vi "SaveTemplatePathToINI.vi"(11 "Template":refnum<class "MetaDataObj.lvclass">) -> ()   [LabVIEW 2016, in "NI_NPW_Project Copying.lvlib"]
uses:
  <resource>/dialog/NewProjectWizard/Project Copying/NI_NPW_Project Copying.lvlib
  <resource>/dialog/NewProjectWizard/MetaDataObj/MetaDataObj.lvclass
  <vilib>/Utility/error.llb/whitespace.ctl
  <resource>/dialog/NewProjectWizard/MetaDataObj/Accessors/Read LocationPath.vi
  <resource>/dialog/NewProjectWizard/MetaDataObj/Accessors/Read Title.vi
  <resource>/dialog/lvconfig.llb/LV Config Read Numeric (I32).vi
panel:
  in  "NewProj.maxNum":string="NewProj.maxNum"
  in  "TemplateTitlesKey":string="NewProj.RecentTitles"
  in  "maxNum Default":i32=10
  in  "TemplatePathsKey":string="NewProj.RecentLocationPaths"
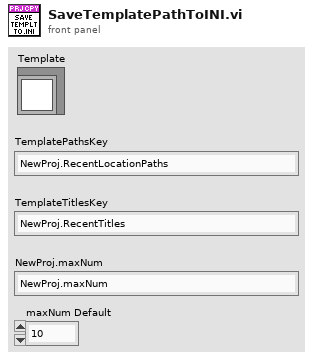
[diagram p1: front panel]
types:
  T1 = typedef "whitespace.ctl" = u16
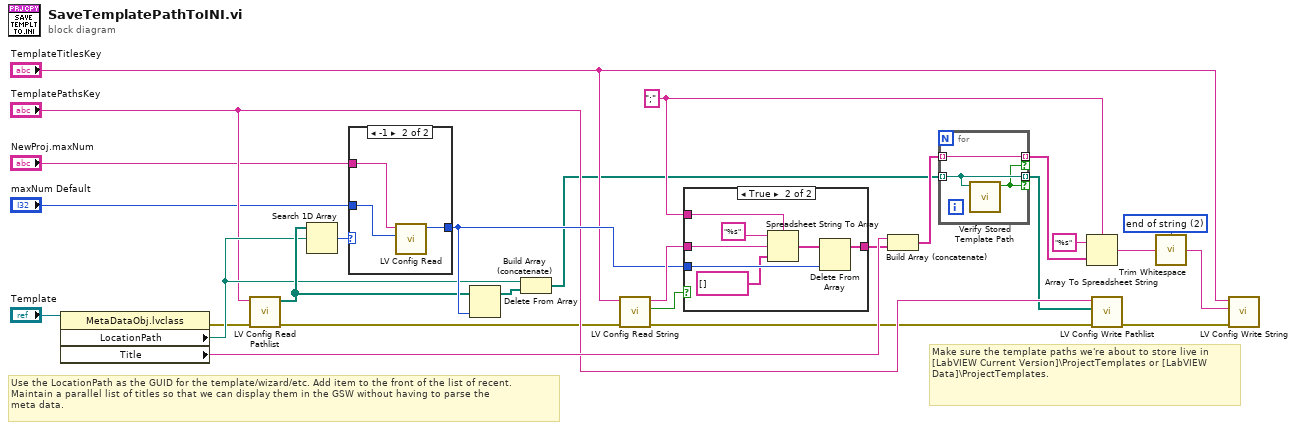
[diagram p0: block diagram]
diagram:
  w13 = T1 2 items=["both", "start of string", "end of string"] ("location (both)")
  w17 = ";" ("delimiter")
  # "Make sure the template paths we're about to store live in [LabVIEW Current Version]\\ProjectTemplates or [LabVIEW Data]\\ProjectTemplates."
  # "Use the LocationPath as the GUID for the template/wizard/etc. Add item to the front of the list of recent.\nMaintain a parallel list of titles so that we can display them in the GSW without having to parse the\nmeta data."
  n1 = property class="MetaDataObj.lvclass"(reference="Template") -> (error out=w18:errorcluster, "LocationPath"=w19:path, "Title"=w20:string)  [unwired: 1 in, 1 out]
  n2 = call <resource>:"LV Config Read Pathlist.vi"("error in"=w18, "key"="TemplatePathsKey") -> ("error out"=w7:errorcluster, "value"=w21:path[])  [unwired: 3 in, 1 out]
  n3 = Search 1D Array(1D array=w21, element=w19) -> (index of element=w27:i32)  [unwired: 1 in]
  n4 = case shown="-1" w27 {
    selector: w27 -> [w28 _]
    tunnel: [w28 w31] -> w23
    tunnel: "NewProj.maxNum" -> [_ w30]
    tunnel: "maxNum Default" -> [_ w29]
    frame Default {
    }
    frame -1 {
      n5 = call-poly <resource>:"LV Config Read.vi"("default value"=w29, "key"=w30) -> ("value"=w31:i32)  [unwired: 3 in, 2 out]
    }
  }
  n6 = Delete From Array(array=w21, index=w23) -> (array with subset deleted=w26:path[])  [unwired: 1 in, 1 out]
  n7 = Build Array (concatenate)(w19, w26) -> (w2:path[])
  n8 = call <resource>:"LV Config Read String.vi"("error in"=w7, "key"="TemplateTitlesKey") -> ("error out"=w6:errorcluster, "found?"=w15:bool, "value"=w24:string)  [unwired: 3 in]
  n9 = case shown="True" w15 {
    tunnel: w24 -> [_ w38]
    tunnel: w23 -> [_ w37]
    tunnel: w17 -> [_ w35]
    tunnel: [_ w33] -> w16
    frame False {
    }
    frame True {
      n10 = Spreadsheet String To Array(delimiter (Tab)=w35, format string="%s", spreadsheet string=w38, array type (2D Dbl)=string[] []) -> (array=w34:string[])
      n11 = Delete From Array(array=w34, index=w37) -> (array with subset deleted=w33:string[])  [unwired: 1 in, 1 out]
    }
  }
  n12 = Build Array (concatenate)(w20, w16) -> (w4:string[])
  n13 = for {
    tunnel: w4 -> [w41] mode=indexing
    tunnel: w2 -> [w40] mode=indexing
    tunnel: [w41] -> w3 mode=indexing if=w39
    tunnel: [w40] -> w1 mode=indexing if=w39
    n14 = call <resource>:"Verify Stored Template Path.vi"("Proposed Template Path"=w40) -> ("Valid Template Path?"=w39:bool)  [unwired: 10 in]
  }
  n15 = Array To Spreadsheet String(delimiter (Tab)=w17, array=w3, 3:"%s" ("format string")) -> (spreadsheet string=w14:string)
  n16 = call <resource>:"LV Config Write Pathlist.vi"("error in (no error)"=w6, "value"=w1, "key"="TemplatePathsKey") -> ("error out"=w5:errorcluster)  [unwired: 4 in]
  n17 = call <vilib>:"Trim Whitespace.vi"("string"=w14, "location (both)"=w13) -> ("trimmed string"=w12:string)
  n18 = call <resource>:"LV Config Write String.vi"("error in (no error)"=w5, "value"=w12, "key"="TemplateTitlesKey") -> ()  [unwired: 4 in, 1 out]
